vi "Test Assert String Ends With.vi"(8 "error in (no error)":errorcluster) -> (0 "error out":errorcluster)   [LabVIEW 2013]
uses:
  classes/Assert/Assert.lvclass
  classes/Test/Test.lvclass
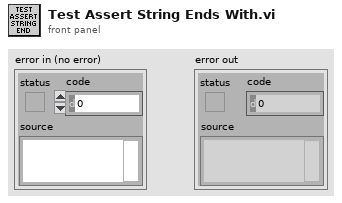
[diagram p1: front panel]
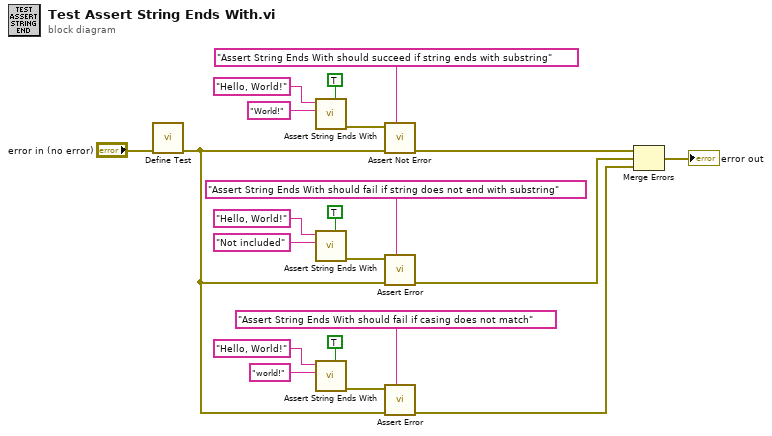
[diagram p0: block diagram]
diagram:
  n1 = call "Define Test.vi"("error in (no error)"="error in (no error)") -> ("error out"=w2:errorcluster)  [unwired: 9 in, 1 out]
  n2 = call "Assert String Ends With.vi"("Assert Only? (F)"=TRUE, "Substring"="World!", "String"="Hello, World!") -> ("error out"=w21:errorcluster)  [unwired: 7 in, 1 out]
  n3 = call "Assert String Ends With.vi"("Assert Only? (F)"=TRUE, "Substring"="Not included", "String"="Hello, World!") -> ("error out"=w9:errorcluster)  [unwired: 7 in, 1 out]
  n4 = call "Assert String Ends With.vi"("Assert Only? (F)"=TRUE, "Substring"="world!", "String"="Hello, World!") -> ("error out"=w7:errorcluster)  [unwired: 7 in, 1 out]
  n5 = call "Assert Not Error.vi"("Label"="Assert String Ends With should succeed if string ends with substring", "error in (no error)"=w2, "Not Error?"=w21) -> ("error out"=w17:errorcluster)  [unwired: 7 in, 1 out]
  n6 = call "Assert Error.vi"("Label"="Assert String Ends With should fail if string does not end with substring", "error in (no error)"=w2, "Error?"=w9) -> ("error out"=w8:errorcluster)  [unwired: 7 in, 1 out]
  n7 = call "Assert Error.vi"("Label"="Assert String Ends With should fail if casing does not match", "error in (no error)"=w2, "Error?"=w7) -> ("error out"=w1:errorcluster)  [unwired: 7 in, 1 out]
  n8 = Merge Errors(w17, w8, w1) -> (→"error out":errorcluster)
